vi "MX100 Close Connection.vi"(8 "error in (no error)":errorcluster, 11 "VISA Refnum in":refnum<visa-resource-name>) -> (0 "error out":errorcluster)   [LabVIEW 2016]
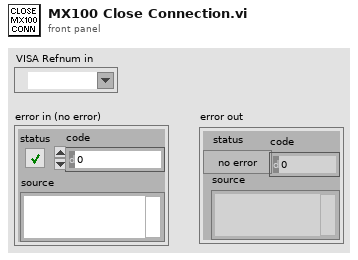
[diagram p1: front panel]
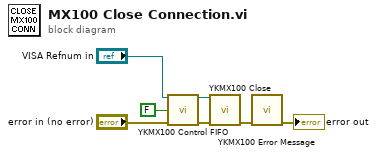
[diagram p0: block diagram]
diagram:
  n1 = call "YKMX100 Control FIFO.vi"("VISA session"="VISA Refnum in", "FIFO (T:Start)"=FALSE, "error in (no error)"="error in (no error)") -> ("dup VISA session"=w2:refnum<visa-resource-name>, "error out"=w3:errorcluster)  [unwired: 10 in, 1 out]
  n2 = call "YKMX100 Close.vi"("VISA session"=w2, "error in (no error)"=w3) -> ("error out"=w6:errorcluster)  [unwired: 13 in]
  n3 = call "YKMX100 Error Message.vi"("error in (no error)"=w6) -> ("error out"=→"error out":errorcluster)  [unwired: 10 in, 4 out]
